vi "matrici_v43.vi"() -> ()   [LabVIEW 2009]
uses:
  <vilib>/Native 3D Graph/xcontrol/3DPC_SurfacePlot.xctl
  <vilib>/Native 3D Graph/classes/Line/Line.lvclass
panel:
  in  "stop":bool
  out "3D Graph":refnum<class "Base Datatype.lvclass">[](xcontrol)
  out "X":dbl=3.326794657762937
  in  "Domeniul de definitie x":dbl(slide)=6.653589315525876 scale=0.5..10.0
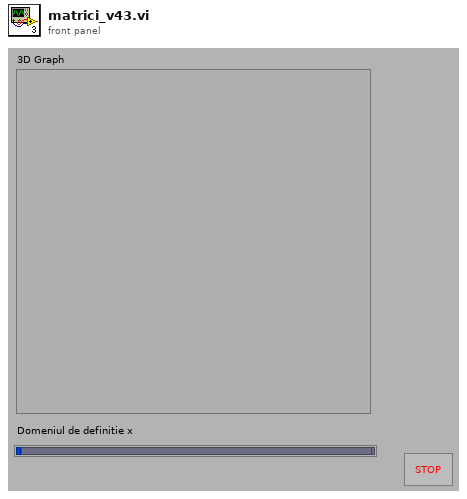
[diagram p1: front panel]
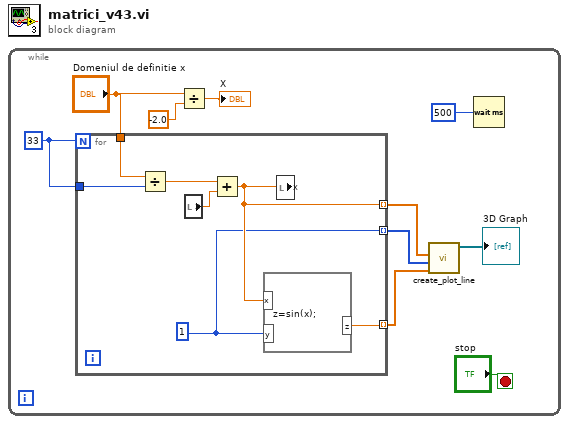
[diagram p0: block diagram]
diagram:
  n1 = while {
    stop <- "stop" stop-if-true
    w9 = 33
    n2 = for {
      N: w9 -> [_]
      tunnel: [w16] -> w3 mode=indexing
      tunnel: w9 -> [w14]
      tunnel: "Domeniul de definitie x" -> [w17]
      tunnel: [w15] -> w1 mode=indexing
      tunnel: [w13] -> w2 mode=indexing
      w13 = 1
      n3 = Divide(x=w17, y=w14) -> (x/y=w11:dbl)
      n4 = local read "X"() -> (w12:dbl)
      n5 = Add(x=w11, y=w12) -> (x+y=w16:dbl)
      n6 = formula code="z=sin(x);"("x"=w16, "y"=w13) -> ("z"=w15:dbl)
      n7 = local write "X"(w16) -> ()
    }
    n8 = Divide(x="Domeniul de definitie x", y=-2.0) -> (x/y=→"X":dbl)
    n9 = call <vilib>:"create_plot_line.vi"("z vector"=w1, "y vector"=w2, "x vector"=w3) -> ("plots out"=→"3D Graph":refnum<class "Base Datatype.lvclass">[])  [unwired: 2 in, 6 out]
    n10 = Wait (ms)(milliseconds to wait=500) -> ()  [unwired: 1 out]
  }
